vi "Maui.Config.ReadApplicationName.vi"(8 "error in (no error)":errorcluster, 11 "Maui.Config in":refnum<class "Maui.Config.lvclass">) -> (0 "error out":errorcluster, 2 "Application Name":string, 3 "Maui.Config out":refnum<class "Maui.Config.lvclass">)   [LabVIEW 2019, in "Maui.Config.lvclass"]
uses:
  Maui.Config.lvclass
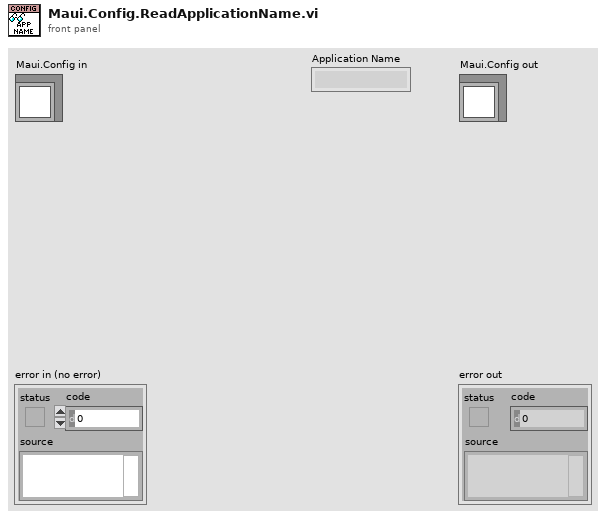
[diagram p1: front panel]
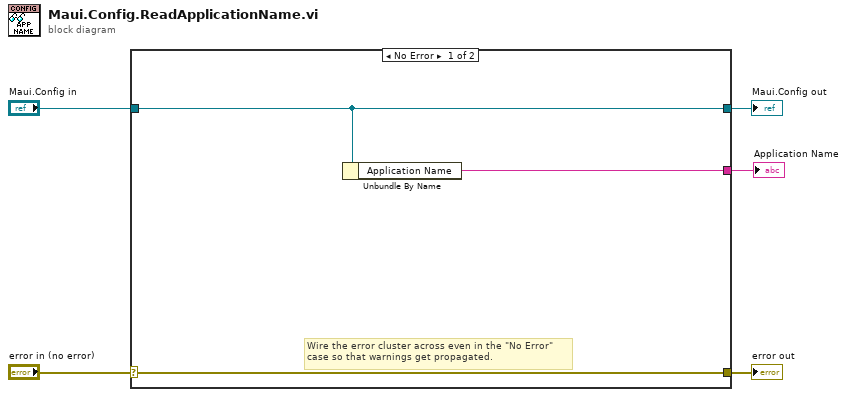
[diagram p0: block diagram]
diagram:
  n1 = case shown="No Error" "error in (no error)" {
    selector: "error in (no error)" -> [w8 w10]
    tunnel: [w8 w10] -> w4
    tunnel: [w7 w9] -> w2
    tunnel: "Maui.Config in" -> [w7 w9]
    tunnel: [w6 _] -> w1
    frame No Error {
      # "Wire the error cluster across even in the \"No Error\"\ncase so that warnings get propagated."
      n2 = Unbundle By Name(w7) -> ("Application Name"=w6:string)
    }
    frame Error {
    }
  }
  "error out" <- w4
  "Maui.Config out" <- w2
  "Application Name" <- w1
